vi "Initialize.vi"(8 "error in (no error)":errorcluster, 11 "Channel in":refnum<class "Channel.lvclass">) -> (0 "error out":errorcluster, 3 "Channel out":refnum<class "Channel.lvclass">)   [LabVIEW 2018, in "Channel.lvclass"]
uses:
  Channel.lvclass
  Channel.lvclass/Channel.ctl
  Image Constructor/Image Constructor.lvclass
  CCDCamera/CCDCamera.lvclass
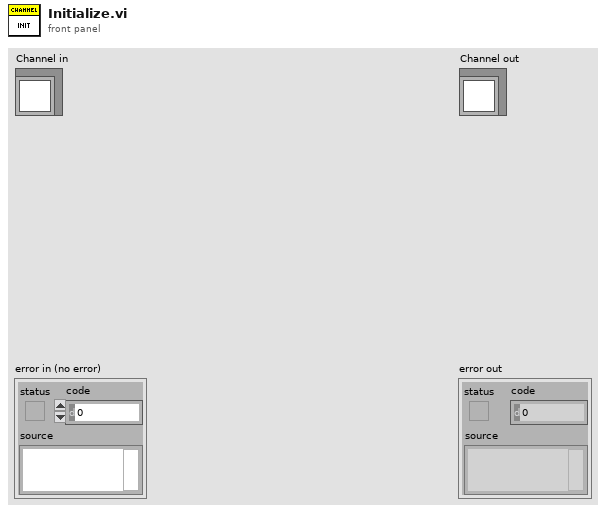
[diagram p1: front panel]
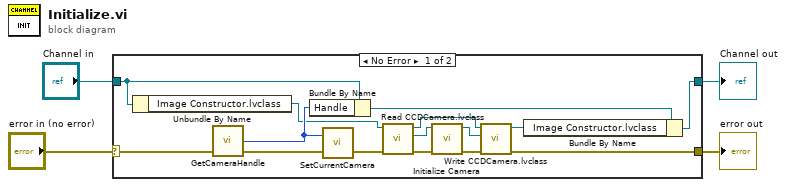
[diagram p0: block diagram]
diagram:
  n1 = case shown="No Error" "error in (no error)" {
    selector: "error in (no error)" -> [w19 w21]
    tunnel: [w8 w21] -> w3
    tunnel: [w7 w20] -> w1
    tunnel: "Channel in" -> [w12 w20]
    frame No Error {
      n2 = Unbundle By Name(w12) -> ("Image Constructor.lvclass"=w16:refnum<class "Image Constructor.lvclass">)
      n3 = call <userlib>:"GetCameraHandle.vi"("error in (no error)"=w19) -> ("error out"=w17:errorcluster, "cameraHandle"=w18:i32)  [unwired: 2 in, 1 out]
      n4 = Bundle By Name(cluster=w12, "Handle"=w18) -> (w11:refnum<class "Channel.lvclass">)
      n5 = call <userlib>:"SetCurrentCamera.vi"("error in (no error)"=w17, "cameraHandle"=w18) -> ("error out"=w15:errorcluster)  [unwired: 1 out]
      n6 = call "Read CCDCamera.lvclass.vi"("error in (no error)"=w15, "Image Constructor in"=w16) -> ("error out"=w13:errorcluster, "CCDCamera.lvclass"=w14:refnum<class "CCDCamera.lvclass">, "Image Constructor out"=w9:refnum<class "Image Constructor.lvclass">)  [unwired: 7 in]
      n7 = call "Initialize Camera.vi"("error in (no error)"=w13, "CCDCamera in"=w14) -> ("error out"=w5:errorcluster, "CCDCamera out"=w6:refnum<class "CCDCamera.lvclass">)  [unwired: 8 in]
      n8 = call "Write CCDCamera.lvclass.vi"("error in (no error)"=w5, "CCDCamera.lvclass"=w6, "Image Constructor in"=w9) -> ("error out"=w8:errorcluster, "Image Constructor out"=w10:refnum<class "Image Constructor.lvclass">)  [unwired: 7 in]
      n9 = Bundle By Name(cluster=w11, "Image Constructor.lvclass"=w10) -> (w7:refnum<class "Channel.lvclass">)
    }
    frame Error {
    }
  }
  "error out" <- w3
  "Channel out" <- w1
